vi "LCD Example.vi"() -> ()   [LabVIEW 2012, in "Phidget LCD.lvlib"]
uses:
  <instrlib>/Phidgets/Phidget LCD/Phidget LCD.lvlib
  <instrlib>/Phidgets/Phidget LCD/Public/LCDStart.vi
  <instrlib>/Phidgets/Phidget LCD/Public/LCDClose.vi
  <instrlib>/Phidgets/Phidget Common/Phidget Common.lvlib
panel:
  out "Screen Height":i32
  out "Screen Width":i32
  out "error out":errorcluster
  in  "error in (no error)":errorcluster
  in  "Device Info":T1={"Serial Number"=-1, "Channel"=0, "Port"=0}
  out "Attached?":bool
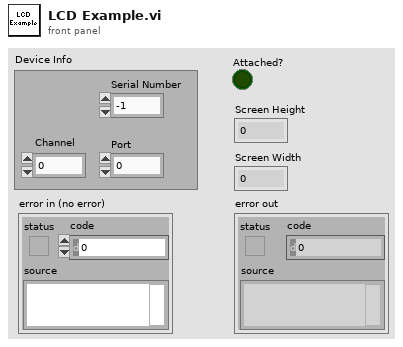
[diagram p1: front panel]
types:
  T1 = cluster{"Serial Number":i32, "Channel":i32, "Port":i32}
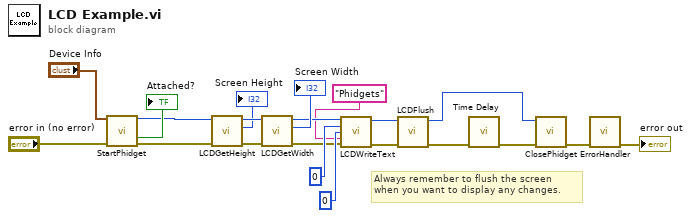
[diagram p0: block diagram]
diagram:
  # "Always remember to flush the screen\nwhen you want to display any changes."
  n1 = call-poly <instrlib>:"StartPhidget.vi"("Device Info"="Device Info", "error in (no error)"="error in (no error)") -> ("Phidget ID"=w6:u64, "Attached?"=→"Attached?":bool, "error out"=w5:errorcluster)  [unwired: 10 in, 1 out]
  n2 = call <instrlib>:"LCDGetHeight.vi"("error in (no error)"=w5, "Device In"=w6) -> ("error out"=w13:errorcluster, "Height"=→"Screen Height":i32, "Device Out"=w12:u64)  [unwired: 7 in]
  n3 = call <instrlib>:"LCDGetWidth.vi"("error in (no error)"=w13, "Device In"=w12) -> ("error out"=w9:errorcluster, "Width"=→"Screen Width":i32, "Device Out"=w8:u64)  [unwired: 7 in]
  n4 = call <instrlib>:"LCDWriteText.vi"("Device In"=w8, "xpos"=0, "ypos"=0, "Text"="Phidgets", "error in (no error)"=w9) -> ("Device Out"=w1:u64, "error out"=w2:errorcluster)  [unwired: 9 in]
  n5 = call <instrlib>:"LCDFlush.vi"("error in (no error)"=w2, "Device In"=w1) -> ("error out"=w4:errorcluster, "Device Out"=w14:u64)  [unwired: 7 in]
  n6 = call "Time Delay"("error in (no error)"=w4) -> ("error out"=w3:errorcluster)  [unwired: 10 in]
  n7 = call-poly <instrlib>:"ClosePhidget.vi"("error in"=w3, "Device In"=w14) -> ("error out"=w18:errorcluster)  [unwired: 9 in]
  n8 = call <instrlib>:"ErrorHandler.vi"("error in"=w18) -> ("error out"=→"error out":errorcluster)  [unwired: 9 in, 1 out]
